vi "ManualControlFlywheels.vi"() -> ()   [LabVIEW 2016]
doc: "The myRIO Project template acquires acceleration data from the onboard accelerometer and displays the changes of acceleration values in a waveform chart."
uses:
  <vilib>/myRIO/Common/Instrument Driver Framework/myRIO v1.0/UART/vis/myRIO v1.0 Close UART.vi
  <vilib>/Utility/error.llb/Error Cluster From Error Code.vi
  <vilib>/myRIO/Common/Instrument Driver Framework/myRIO v1.0/PWM/vis/myRIO v1.0 Write PWM.vi
  <vilib>/myRIO/Common/Instrument Driver Framework/Utilities/vis/FPGA Ref Manager.vi
  <vilib>/myRIO/Common/Instrument Driver Framework/myRIO v1.0/myRIO v1.0 Reset FPGA.vi
  <vilib>/myRIO/Common/Instrument Driver Framework/myRIO v1.0/IRQ/vis/myRIO v1.0 IRQ Info FGV.vi
  <vilib>/myRIO/Common/Instrument Driver Framework/myRIO v1.0/IRQ/vis/myRIO v1.0 Timer IRQ Info FGV.vi
  <vilib>/myRIO/Common/Instrument Driver Framework/myRIO v1.0/IRQ/vis/myRIO v1.0 ISR Agent.vi
  <vilib>/myRIO/Instrument Drivers/Utilities/Utilities.lvlib
  <vilib>/myRIO/Instrument Drivers/Onboard IO/PWM/PWM.lvlib
panel:
  out "Boolean 3":bool
  out "Boolean 2":bool
  out "Boolean":bool
  out "Numeric":dbl
  in  "Duty Cycle 2":dbl min=0.0 max=0.08
  in  "Duty Cycle 1":dbl min=0.0 max=0.08
  in  "Duty Cycle 0":dbl min=0.0 max=0.08
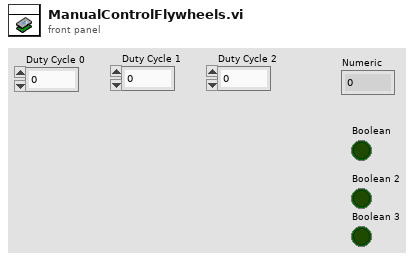
[diagram p1: front panel]
types:
  T1 = typedef "PWM.lvlib/PWM Reference.ctl" = cluster{"myRIO Reference":T2, "PWM Channels Enum":T6, "PWM Configuration":T7}
  T2 = typedef "myRIO Generic Hardware Reference.ctl" = cluster{"myRIO Model":T3, "myRIO Hardware Reference":T4}
  T3 = typedef "Hardware Version Enum.ctl" = enum16{"Unknown", "myRIO-1900", "myRIO-1950", "roboRIO", "NI ELVIS RIO CM"}
  T4 = typedef "myRIO v1.0 Reference.ctl" = cluster{"Generic FPGA Reference":T5, "Allow multiple opens":bool}
  T5 = typedef "Generic FPGA Reference.ctl" = refnum<k20>
  T6 = typedef "PWM Channels Enum.ctl" = enum16{"Not Connected", "C/PWM0", "C/PWM1", "A/PWM0", "A/PWM1", "A/PWM2", "B/PWM0", "B/PWM1", "B/PWM2", "PWM/PWM0", "PWM/PWM1", "PWM/PWM2", "PWM/PWM3", "PWM/PWM4", "PWM/PWM5", "PWM/PWM6", "PWM/PWM7", "PWM/PWM8", "PWM/PWM9"}
  T7 = typedef "PWM.lvlib/PWM Configuration.ctl" = cluster{"Frequency":dbl, "Duty Cycle":dbl}
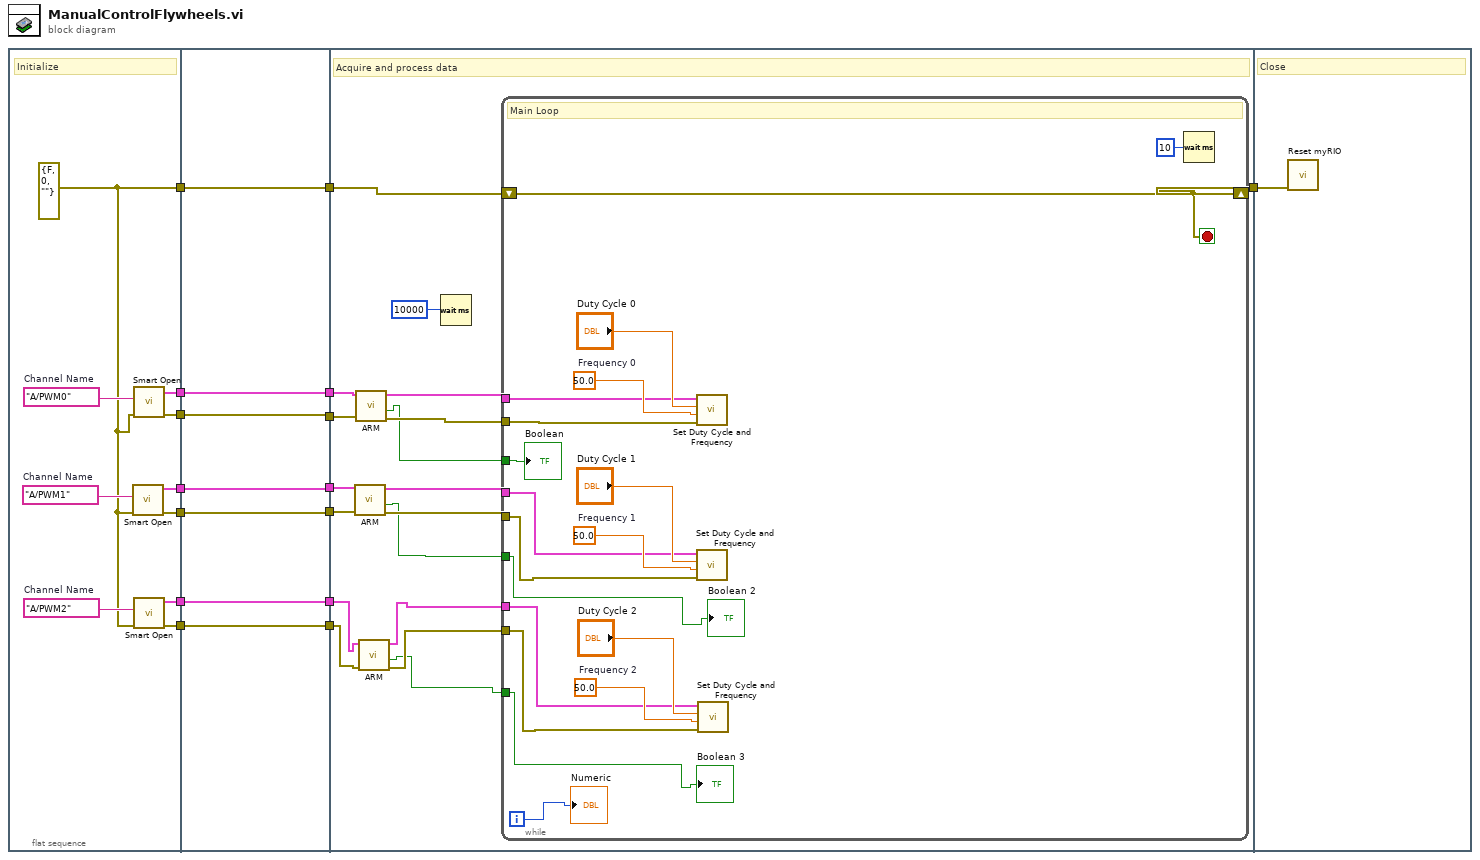
[diagram p0: block diagram]
diagram:
  n1 = flat-sequence {
    tunnel: [w20] -> w14
    tunnel: [w25] -> w12
    tunnel: [w24] -> w11
    tunnel: [w19] -> w8
    tunnel: [w18] -> w7
    tunnel: [w17] -> w6
    tunnel: [w16] -> w5
    tunnel: w14 -> [w32]
    tunnel: [w32] -> w13
    tunnel: w12 -> [w31]
    tunnel: w11 -> [w30]
    tunnel: [w31] -> w10
    tunnel: [w30] -> w9
    tunnel: w8 -> [w29]
    tunnel: w7 -> [w28]
    tunnel: w6 -> [w27]
    tunnel: w5 -> [w26]
    tunnel: [w29] -> w4
    tunnel: [w28] -> w3
    tunnel: [w27] -> w2
    tunnel: [w26] -> w1
    tunnel: w13 -> [w50]
    tunnel: [w49] -> w15
    tunnel: w10 -> [w40]
    tunnel: w9 -> [w39]
    tunnel: w4 -> [w44]
    tunnel: w3 -> [w43]
    tunnel: w2 -> [w48]
    tunnel: w1 -> [w47]
    tunnel: w15 -> [w69]
    frame #0 {
      w21 = tag "A/PWM2"  # Channel Name
      w22 = tag "A/PWM1"  # Channel Name
      w23 = tag "A/PWM0"  # Channel Name
      w20 = errorcluster {"status"=FALSE, "code"=0, "source"=""} ("error in (no error)")
      # "Initialize"
      n2 = call <vilib>:"Smart Open.vi"("error in (no error)"=w20, "Channel Name"=w22) -> ("error out"=w18:errorcluster, "PWM Ref Out"=w19:T1)  [unwired: 8 in]
      n3 = call <vilib>:"Smart Open.vi"("error in (no error)"=w20, "Channel Name"=w23) -> ("error out"=w24:errorcluster, "PWM Ref Out"=w25:T1)  [unwired: 8 in]
      n4 = call <vilib>:"Smart Open.vi"("error in (no error)"=w20, "Channel Name"=w21) -> ("error out"=w16:errorcluster, "PWM Ref Out"=w17:T1)  [unwired: 8 in]
    }
    frame #1 {
    }
    frame #2 {
      # "Acquire and process data"
      n5 = call "ARM.vi"("error in (no error)"=w43, "PWM Ref in"=w44) -> ("error out"=w41:errorcluster, "Boolean"=w35:bool, "PWM Ref out"=w42:T1)  [unwired: 7 in]
      n6 = call "ARM.vi"("error in (no error)"=w39, "PWM Ref in"=w40) -> ("error out"=w37:errorcluster, "Boolean"=w34:bool, "PWM Ref out"=w38:T1)  [unwired: 7 in]
      n7 = call "ARM.vi"("error in (no error)"=w47, "PWM Ref in"=w48) -> ("error out"=w45:errorcluster, "Boolean"=w36:bool, "PWM Ref out"=w46:T1)  [unwired: 7 in]
      n8 = Wait (ms)(milliseconds to wait=u32 10000) -> ()  [unwired: 1 out]
      n9 = while {
        shift-right: [w67] -> w49
        shift-left: w50 -> [w67]
        tunnel: w37 -> [w58]
        tunnel: w38 -> [w59]
        tunnel: w42 -> [w57]
        tunnel: w41 -> [w56]
        tunnel: w46 -> [w55]
        tunnel: w45 -> [w54]
        tunnel: w36 -> [w51]
        tunnel: w35 -> [w52]
        tunnel: w34 -> [w53]
        i -> [w66]
        stop <- w67 stop-if-true
        w64 = 50.0  # Frequency 0
        w61 = 50.0  # Frequency 2
        w63 = 50.0  # Frequency 1
        # "Main Loop"
        n10 = call <vilib>:"Set Duty Cycle and Frequency.vi"("error in (no error)"=w58, "Frequency [Hz]"=w64, "Duty Cycle"="Duty Cycle 0", "PWM Ref In"=w59) -> ()  [unwired: 5 in, 2 out]
        n11 = call <vilib>:"Set Duty Cycle and Frequency.vi"("error in (no error)"=w56, "Frequency [Hz]"=w63, "Duty Cycle"="Duty Cycle 1", "PWM Ref In"=w57) -> ()  [unwired: 5 in, 2 out]
        n12 = call <vilib>:"Set Duty Cycle and Frequency.vi"("error in (no error)"=w54, "Frequency [Hz]"=w61, "Duty Cycle"="Duty Cycle 2", "PWM Ref In"=w55) -> ()  [unwired: 5 in, 2 out]
        n13 = Wait (ms)(milliseconds to wait=u32 10) -> ()  [unwired: 1 out]
        "Numeric" <- w66
        "Boolean" <- w53
        "Boolean 2" <- w52
        "Boolean 3" <- w51
      }
    }
    frame #3 {
      # "Close"
      n14 = call <vilib>:"Reset myRIO.vi"("error in (no error)"=w69) -> ()  [unwired: 10 in, 1 out]
    }
  }
